vi "CTRE_CANifier_SetLEDOutput.vi"(8 "error in":errorcluster, 9 "LEDChannel":T2, 10 "Percent Output":dbl min=0.0 max=1.0 step=0.01 format="%#_13g", 11 "CANifierDevRef":T1) -> (0 "error out":errorcluster, 3 "CANifierDevRef":T1)   [LabVIEW 2016]
uses:
  <vilib>/Rock Robotics/WPI/ThirdParty/Sensors/CANifier/CTRE_CANifier_LEDChannel.ctl
  <vilib>/Rock Robotics/WPI/ThirdParty/Sensors/CANifier/CTRE_CANifier_DeviceRef.ctl
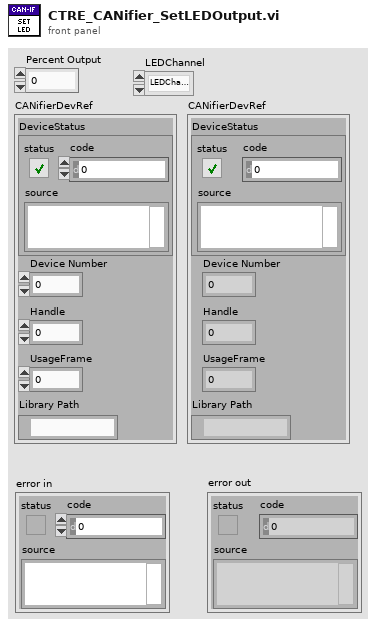
[diagram p1: front panel]
types:
  T1 = typedef "CTRE_CANifier_DeviceRef.ctl" = cluster{"DeviceStatus":errorcluster, "Device Number":u8, "Handle":u64, "UsageFrame":u32, "Library Path":path}
  T2 = typedef "CTRE_CANifier_LEDChannel.ctl" = enum32{"LEDChannelA", "LEDChannelB", "LEDChannelC"}
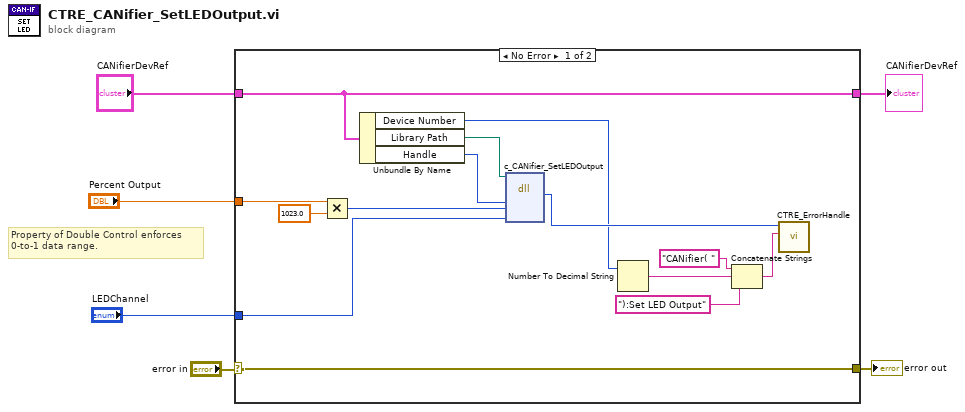
[diagram p0: block diagram]
diagram:
  # "Property of Double Control enforces\n0-to-1 data range."
  n1 = case shown="No Error" "error in" {
    selector: "error in" -> [w20 w22]
    tunnel: [w20 w22] -> w5
    tunnel: "LEDChannel" -> [w13 _]
    tunnel: "Percent Output" -> [w19 _]
    tunnel: "CANifierDevRef" -> [w17 w21]
    tunnel: [w17 w21] -> w1
    frame No Error {
      n2 = Multiply(x=w19, y=1023.0) -> (x*y=w14:u32)
      n3 = Unbundle By Name(w17) -> ("Device Number"=w8:u8, "Library Path"=w16:path, "Handle"=w15:u64)
      n4 = dll-call lib="?" fn="c_CANifier_SetLEDOutput"(path in=w16, "handle"=w15, "dutyCycle"=w14, "ledChannel"=w13) -> ("CTR_Code"=w12:i8)  [unwired: 5 in, 2 out]
      n5 = Number To Decimal String(number=w8) -> (decimal integer string=w11:string)  [unwired: 1 in]
      n6 = Concatenate Strings("CANifier( " ("string"), w11, "):Set LED Output" ("string")) -> (w7:string)
      n7 = call <vilib>:"CTRE_ErrorHandle.vi"("origin"=w7, "code"=w12) -> ()  [unwired: 9 in, 1 out]
    }
    frame Error {
    }
  }
  "error out" <- w5
  "CANifierDevRef" <- w1
